vi "Determine VISA interface to open.vi"(9 "Port (7020)":string, 10 "IP Address":string, 11 "VISA resource name":refnum<visa-resource-name>) -> (3 "VISA resource name out":refnum<visa-resource-name>)   [LabVIEW 2019, in "Mercury iXX.lvlib"]
uses:
  Mercury iXX.lvlib
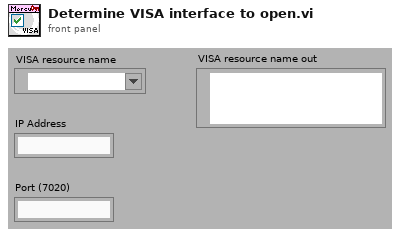
[diagram p1: front panel]
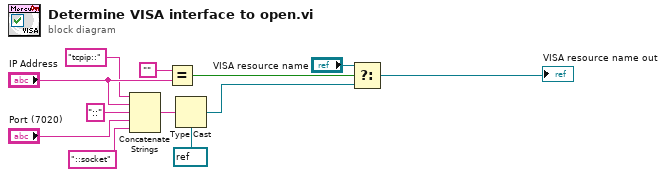
[diagram p0: block diagram]
diagram:
  n1 = Concatenate Strings("tcpip::" ("string"), "IP Address", "::" ("string"), "Port (7020)", "::socket" ("string")) -> (w5:string)
  n2 = Equal?(x="", y="IP Address") -> (x = y?=w10:bool)
  n3 = Type Cast(type=refnum<visa-resource-name> refnum ("VISA resource name"), x=w5) -> (*(type *) &x=w12:refnum<visa-resource-name>)
  n4 = Select(t="VISA resource name", s=w10, f=w12) -> (s? t:f=→"VISA resource name out":refnum<visa-resource-name>)
